vi "writeParameterXML.vi"(8 "error in (no error)":errorcluster, 11 "ScriptEvent in":refnum<class "ScriptEvent.lvclass">) -> (0 "error out":errorcluster, 3 "ScriptEvent out":refnum<class "ScriptEvent.lvclass">)   [LabVIEW 2011, in "Tools.lvlib" / "Scripting.lvlib" / "ScriptEvent.lvclass"]
uses:
  ScriptEvent.lvclass
  xmlNode/xmlNode.lvclass
panel:
  in  "xmlArray":refnum<class "xmlNode.lvclass">[](array[class])
  out "xmlArray":refnum<class "xmlNode.lvclass">[](array[class])
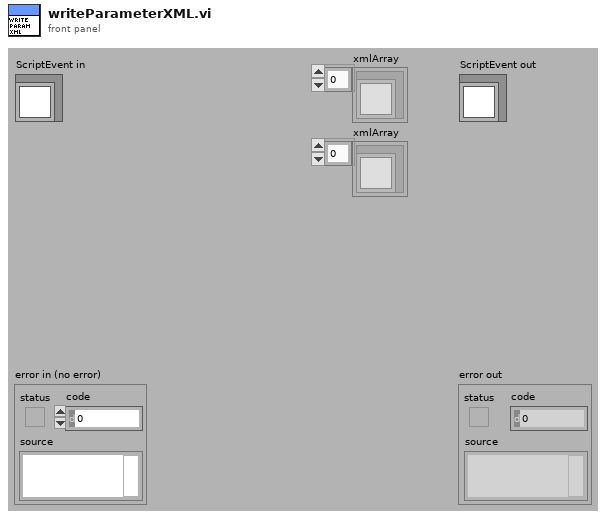
[diagram p1: front panel]
types:
  T1 = cluster{"parameter_name":string, "parameter_value":string, "type":enum16{"time", "time_difference", "value", "frequency", "phase", "ramp_time", "value_step", "time_step", "number_of_steps", "start_value", "end_value", "start_freq", "start_amp", "start_phase", "end_freq", "end_amp", "end_phase"}}[]
  T2 = enum16{"time", "time_difference", "value", "frequency", "phase", "ramp_time", "value_step", "time_step", "number_of_steps", "start_value", "end_value", "start_freq", "start_amp", "start_phase", "end_freq", "end_amp", "end_phase"}
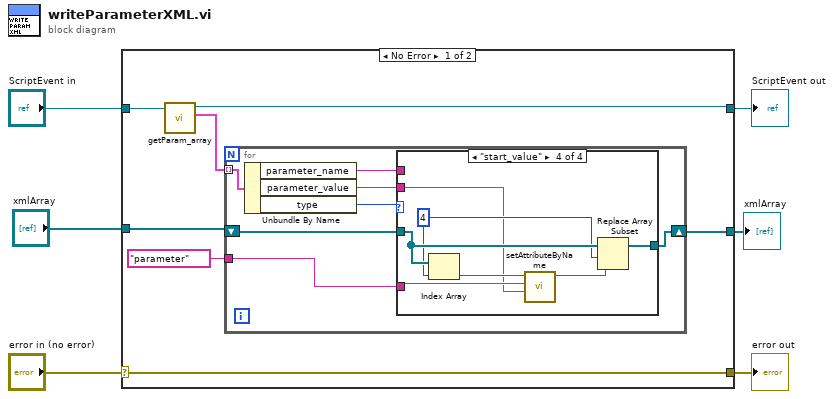
[diagram p0: block diagram]
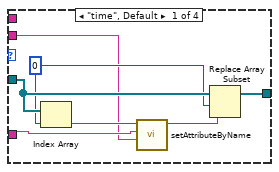
[diagram p2: hidden frame]
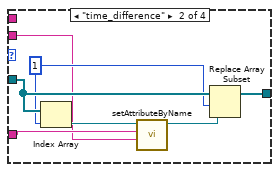
[diagram p3: hidden frame]
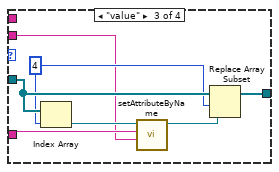
[diagram p4: hidden frame]
diagram:
  n1 = case shown="No Error" "error in (no error)" {
    selector: "error in (no error)" -> [w9 w50]
    tunnel: [w9 w50] -> w5
    tunnel: [w10 w49] -> w3
    tunnel: "ScriptEvent in" -> [w11 w49]
    tunnel: [w8 _] -> w2
    tunnel: "xmlArray" -> [w7 _]
    frame No Error {
      n2 = call "getParam_array.vi"("ScriptEvent in"=w11) -> ("param_array"=w12:T1, "ScriptEvent out"=w10:refnum<class "ScriptEvent.lvclass">)  [unwired: 8 in, 1 out]
      n3 = for {
        tunnel: w12 -> [w20] mode=indexing
        shift-right: [w15] -> w8
        shift-left: w7 -> [w18]
        tunnel: "parameter" -> [w14]
        n4 = Unbundle By Name(w20) -> ("parameter_name"=w17:string, "parameter_value"=w16:string, "type"=w19:T2)
        n5 = case shown="\"start_value\"" w19 {
          tunnel: w18 -> [w25 w32 w39 w46]
          tunnel: w17 -> [_ _ _ _]
          tunnel: w16 -> [w21 w28 w35 w42]
          tunnel: [w23 w30 w37 w44] -> w15
          tunnel: w14 -> [w22 w29 w36 w43]
          frame "time", Default {
            w24 = 0
            n6 = Index Array(array=w25, index=w24) -> (element=w27:refnum<class "xmlNode.lvclass">)
            n7 = call-dynamic "setAttributeByName.vi"("attributeValue"=w21, "attributeName"=w22, "xmlNode in"=w27) -> ("xmlNode out"=w26:refnum<class "xmlNode.lvclass">)  [unwired: 7 in, 1 out]
            n8 = Replace Array Subset(array=w25, new element=w26, index=w24) -> (w23:refnum<class "xmlNode.lvclass">[])
          }
          frame "time_difference" {
            w31 = 1
            n9 = Index Array(array=w32, index=w31) -> (element=w34:refnum<class "xmlNode.lvclass">)
            n10 = call-dynamic "setAttributeByName.vi"("attributeValue"=w28, "attributeName"=w29, "xmlNode in"=w34) -> ("xmlNode out"=w33:refnum<class "xmlNode.lvclass">)  [unwired: 7 in, 1 out]
            n11 = Replace Array Subset(array=w32, new element=w33, index=w31) -> (w30:refnum<class "xmlNode.lvclass">[])
          }
          frame "value" {
            w38 = 4
            n12 = Index Array(array=w39, index=w38) -> (element=w41:refnum<class "xmlNode.lvclass">)
            n13 = call-dynamic "setAttributeByName.vi"("attributeValue"=w35, "attributeName"=w36, "xmlNode in"=w41) -> ("xmlNode out"=w40:refnum<class "xmlNode.lvclass">)  [unwired: 7 in, 1 out]
            n14 = Replace Array Subset(array=w39, new element=w40, index=w38) -> (w37:refnum<class "xmlNode.lvclass">[])
          }
          frame "start_value" {
            w45 = 4
            n15 = Index Array(array=w46, index=w45) -> (element=w48:refnum<class "xmlNode.lvclass">)
            n16 = call-dynamic "setAttributeByName.vi"("attributeValue"=w42, "attributeName"=w43, "xmlNode in"=w48) -> ("xmlNode out"=w47:refnum<class "xmlNode.lvclass">)  [unwired: 7 in, 1 out]
            n17 = Replace Array Subset(array=w46, new element=w47, index=w45) -> (w44:refnum<class "xmlNode.lvclass">[])
          }
        }
      }
    }
    frame Error {
    }
  }
  "error out" <- w5
  "ScriptEvent out" <- w3
  "xmlArray" <- w2
